vi "ReadDigitalOutput.vi"(8 "error in (no error)":errorcluster, 11 "TesteractHAL_DigitalIO In":refnum<class "TesteractHAL_DigitalOutput_EthernetModbus.lvclass">) -> (0 "error out":errorcluster, 1 "Tristate":bool, 2 "data":bool, 3 "TesteractHAL_DigitalIO Out":refnum<class "TesteractHAL_DigitalOutput_EthernetModbus.lvclass">)   [LabVIEW 2017, in "TesteractHAL_DigitalOutput_EthernetModbus.lvlib" / "TesteractHAL_DigitalOutput_EthernetModbus.lvclass"]
doc: "Read a single digital bool."
uses:
  TesteractHAL_DigitalOutput_EthernetModbus.lvclass
  C:/Program Files (x86)/Testeract/HWLib/HAL/Device/TesteractHAL_Device.lvlibp/TesteractHAL_Device.lvclass
  TesteractHAL_DigitalOutput_EthernetModbus.lvclass/TesteractHAL_DigitalOutput_EthernetModbus.ctl
  Program Files (x86)/Testeract/HWLib/HAL/Device/TesteractHAL_Device.lvlibp/ReadConnectionAlias.vi
  Drivers/NIModbus/NI Modbus.llb/MB Ethernet Master Query Read Coils (poly).vi
  Program Files (x86)/Testeract/TCPConnectionManager/Testeract_TCPConnectionManager.lvlibp/Testeract_TCPConnectionManager.lvclass
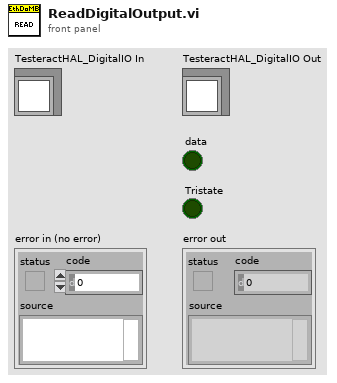
[diagram p1: front panel]
types:
  T1 = typedef "Testeract_TCPConnectionManager.lvlibp/Semaphore RefNum" = refnum<k1>
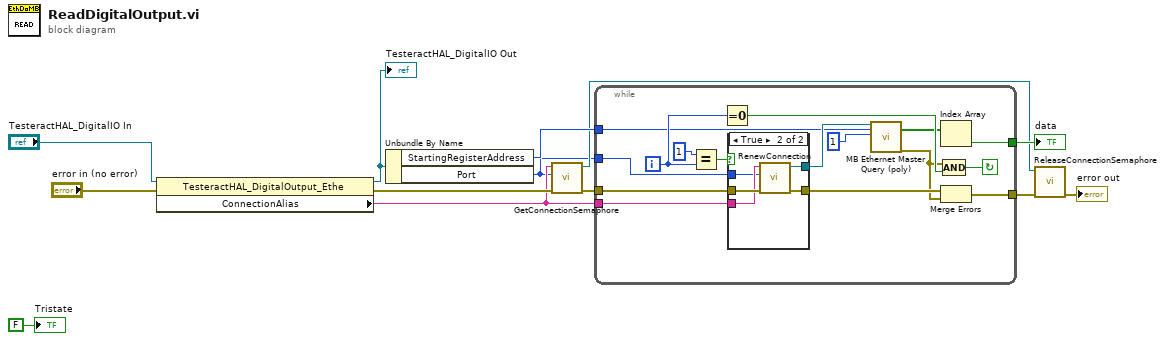
[diagram p0: block diagram]
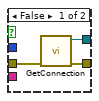
[diagram p2: hidden frame]
diagram:
  n1 = property class="TesteractHAL_DigitalOutput_Ethe"(reference="TesteractHAL_DigitalIO In", error in="error in (no error)") -> (reference out=w10:refnum<class "TesteractHAL_DigitalOutput_EthernetModbus.lvclass">, error out=w5:errorcluster, "ConnectionAlias"=w2:string)
  "TesteractHAL_DigitalIO Out" <- w10
  n2 = Unbundle By Name(w10) -> ("StartingRegisterAddress"=w13:u16, "Port"=w1:u16)
  n3 = call "GetConnectionSemaphore.vi"("error in (no error)"=w5, "Port"=w1, "IPAddress"=w2) -> ("error out"=w4:errorcluster, "Semaphore Ref"=w3:T1)  [unwired: 7 in]
  n4 = while {
    tunnel: w2 -> [w29]
    tunnel: w4 -> [w28]
    tunnel: [w21] -> w7
    tunnel: w13 -> [w18]
    tunnel: w1 -> [w17]
    tunnel: [w14] -> w9
    i -> [w23]
    stop <- w24 continue-if-true
    n5 = Equal?(x=1, y=w23) -> (x = y?=w26:bool)
    n6 = Equal To 0?(x=w23) -> (x = 0?=w22:bool)
    n7 = case shown="True" w26 {
      tunnel: w29 -> [_ w34]
      tunnel: w28 -> [w32 w37]
      tunnel: [w30 w35] -> w19
      tunnel: [w31 w36] -> w25
      tunnel: w17 -> [_ w33]
      frame False {
        n8 = call "GetConnection.vi"("error in (no error)"=w32) -> ("error out"=w31:errorcluster, "Connection ID"=w30:refnum<k5>)  [unwired: 9 in]
      }
      frame True {
        n9 = call "RenewConnection.vi"("error in (no error)"=w37, "Port"=w33, "IPAddress"=w34) -> ("error out"=w36:errorcluster, "Connection ID"=w35:refnum<k5>)  [unwired: 7 in]
      }
    }
    n10 = call-poly "MB Ethernet Master Query (poly).vi"("TCP Connection Refnum in"=w19, "Starting Address"=w18, "Quantity"=u16 1) -> ("Coils"=w16:bool[], "error out"=w20:errorcluster)  [unwired: 2 in, 13 out]
    n11 = Index Array(array=w16) -> (element=w14:bool)  [unwired: 1 in]
    n12 = Merge Errors(w25, w20) -> (w21:errorcluster)
    n13 = Compound Arithmetic op=AND(w20, w22) -> (w24:bool)
  }
  "data" <- w9
  n14 = call "ReleaseConnectionSemaphore.vi"("error in (no error)"=w7, "Semaphore Refnum"=w3) -> ("error out"=→"error out":errorcluster)  [unwired: 9 in]
  "Tristate" <- FALSE ("Tristate")
